vi "ATF-DI Search Channel.vi"(11 "DI Data":digitalwaveform[](array[waveform])) -> (3 "Array 2":bool[](array[boolean]))   [LabVIEW 2022 SP3]
uses:
  <vilib>/Waveform/DTblOps.llb/DTbl Digital to Boolean Array.vi
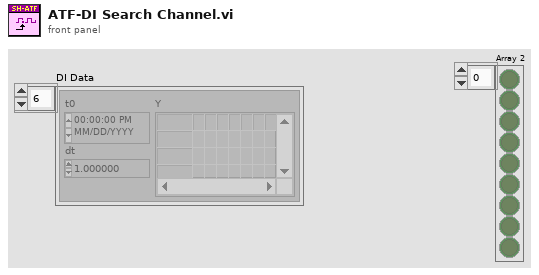
[diagram p1: front panel]
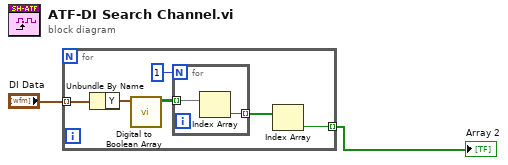
[diagram p0: block diagram]
diagram:
  n1 = for {
    tunnel: "DI Data" -> [w5] mode=indexing
    tunnel: [w3] -> w1 mode=indexing
    n2 = Unbundle By Name(w5) -> ("Y"=w6:digitaldata)
    n3 = call-poly <vilib>:"Digital to Boolean Array.vi"("digital data"=w6) -> ("boolean array"=w7:bool[][])  [unwired: 9 in, 1 out]
    n4 = for {
      N: 1 -> [_]
      tunnel: w7 -> [w10] mode=indexing
      tunnel: [w9] -> w4 mode=indexing
      n5 = Index Array(array=w10) -> (element=w9:bool)  [unwired: 1 in]
    }
    n6 = Index Array(array=w4) -> (element=w3:bool)  [unwired: 1 in]
  }
  "Array 2" <- w1
